vi "Part 2.vi"(11 "Input":string) -> (3 "Output":i32)   [LabVIEW 2021]
panel:
  out "Waveform Graph":i32[](graph)
  out "min index(es)":i32
  # "94813700"
  # "94813675"
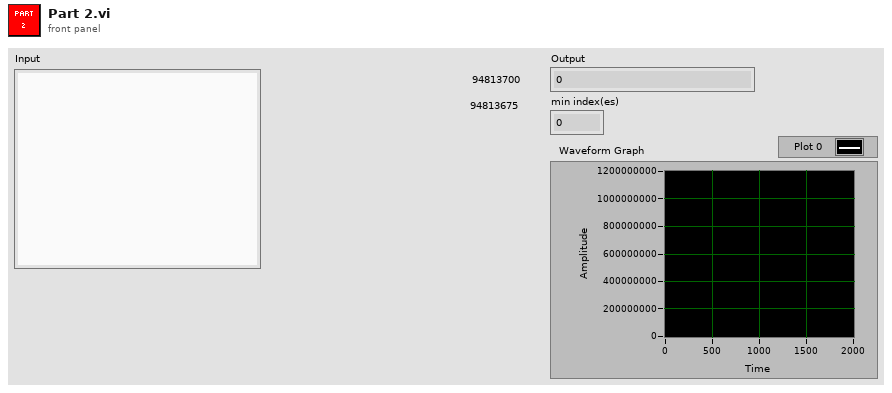
[diagram p1: front panel]
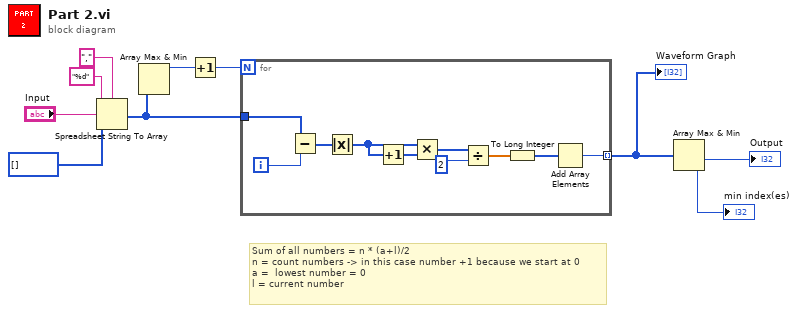
[diagram p0: block diagram]
diagram:
  # "Sum of all numbers = n * (a+l)/2\nn = count numbers -> in this case number +1 because we start at 0\na =  lowest number = 0\nl = current number"
  n1 = Spreadsheet String To Array(delimiter (Tab)=",", format string="%d", spreadsheet string="Input", array type (2D Dbl)=i32[] []) -> (array=w3:i32[])
  n2 = Array Max & Min(array=w3) -> (max value=w4:i32)  [unwired: 3 out]
  n3 = Increment(x=w4) -> (x+1=w2:i32)
  n4 = for {
    N: w2 -> [_]
    tunnel: w3 -> [w20]
    tunnel: [w18] -> w5 mode=indexing
    i -> [w13]
    n5 = Subtract(x=w20, y=w13) -> (x-y=w19:i32[])
    n6 = Absolute Value(x=w19) -> (abs(x)=w12:i32[])
    n7 = Increment(x=w12) -> (x+1=w17:i32[])
    n8 = Multiply(x=w12, y=w17) -> (x*y=w16:i32[])
    n9 = Divide(x=w16, y=2) -> (x/y=w14:dbl[])
    n10 = To Long Integer(number=w14) -> (32bit integer=w11:i32[])
    n11 = Add Array Elements(numeric array=w11) -> (sum=w18:i32)
  }
  "Waveform Graph" <- w5
  n12 = Array Max & Min(array=w5) -> (min value=→"Output":i32, min index (indices)=→"min index(es)":i32)  [unwired: 2 out]
